vi "Parameters.vi"() -> ()   [LabVIEW 2020, in "Parameters Lib.lvlib"]
uses:
  Parameters Lib.lvlib
  Database Lib.lvlib
panel:
  in  "Reject Based on":string(combo)
  in  "Maximum Area (mm)":i32
  in  "Maximum Length (mm)":i32
  in  "Maximum Width (mm)":i32
  in  "Close":bool
  # "Parameters"
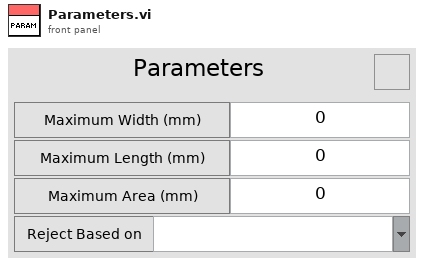
[diagram p1: front panel]
types:
  T1 = cluster{"Maximum Width (mm)":i32, "Maximum Length (mm)":i32, "Maximum Area (mm)":i32, "Reject Based on":string}
  T2 = cluster{"Maximum Width (mm)":i32, "Maximum Length (mm)":i32, "Maximum Area (mm)":i32, "Reject Based on":string}[]
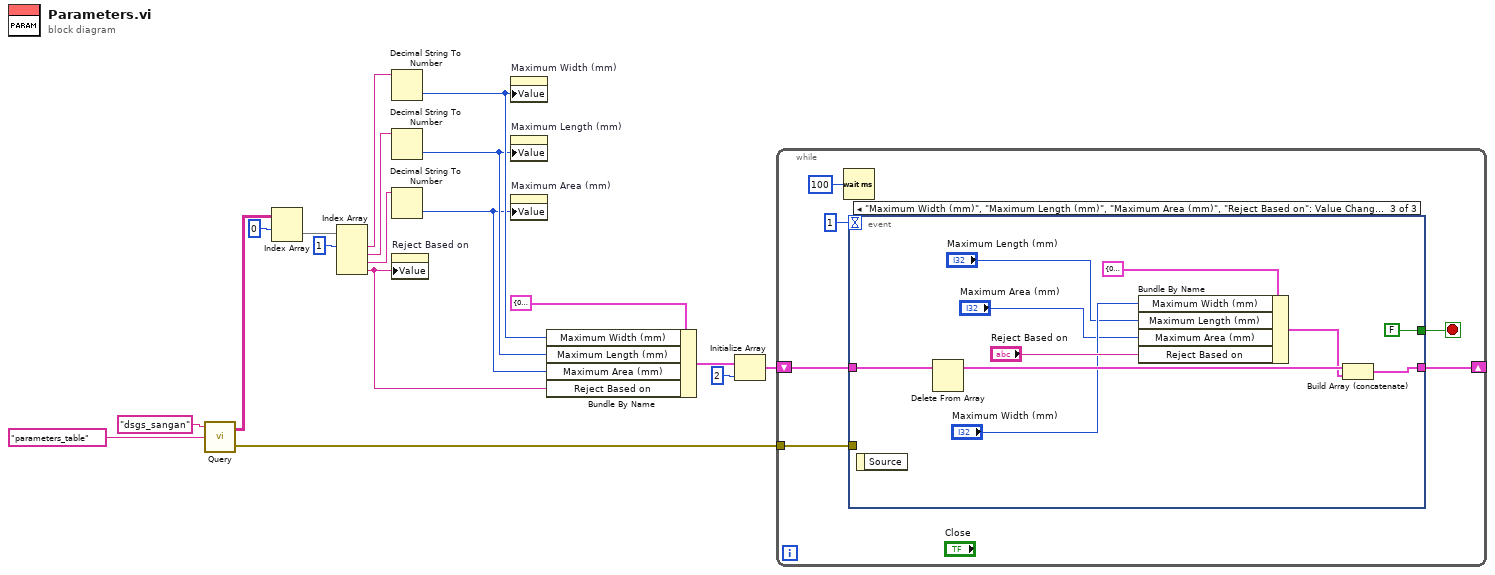
[diagram p0: block diagram]
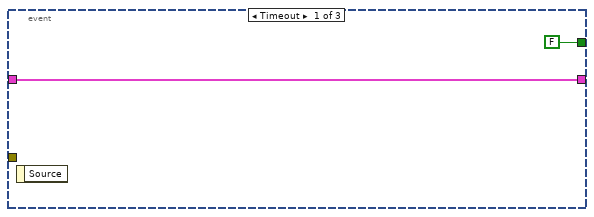
[diagram p2: hidden frame]
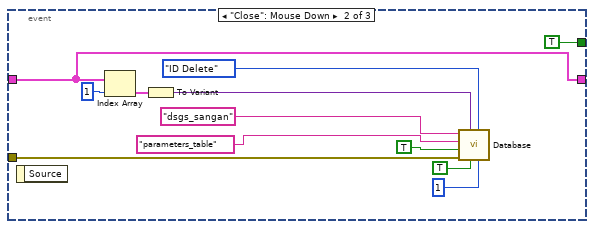
[diagram p3: hidden frame]
diagram:
  n1 = call "Query.vi"("Table Name"="parameters_table" ("Table"), "Connection Name"="dsgs_sangan") -> ("Error out"=w14:errorcluster, "data"=w13:string[][])  [unwired: 2 in]
  n2 = Index Array(array=w13, index (row)=0) -> (element=w11:string[])  [unwired: 1 in]
  n3 = Index Array(array=w11, index #1=1 ("index")) -> (element #1=w8:string, element #2=w6:string, element #3=w7:string, element #4=w1:string)  [unwired: 3 in]
  n4 = Decimal String To Number(string=w8) -> (number=w4:i32)  [unwired: 2 in, 1 out]
  n5 = Decimal String To Number(string=w6) -> (number=w3:i32)  [unwired: 2 in, 1 out]
  n6 = Decimal String To Number(string=w7) -> (number=w2:i32)  [unwired: 2 in, 1 out]
  n7 = property on="Reject Based on" class="CmbBox"("Value"=w1) -> ()  [unwired: 2 in, 2 out]
  n8 = property on="Maximum Width (mm)" class="DigNum (strict)"("Value"=w4) -> ()  [unwired: 2 in, 2 out]
  n9 = property on="Maximum Length (mm)" class="DigNum (strict)"("Value"=w3) -> ()  [unwired: 2 in, 2 out]
  n10 = property on="Maximum Area (mm)" class="DigNum (strict)"("Value"=w2) -> ()  [unwired: 2 in, 2 out]
  n11 = Bundle By Name(cluster=T1 {"Maximum Width (mm)"=0, "Maximum Length (mm)"=0, "Maximum Area (mm)"=0, "Reject Based on"=""}, "Maximum Width (mm)"=w4, "Maximum Length (mm)"=w3, "Maximum Area (mm)"=w2, "Reject Based on"=w1) -> (w9:T1)
  n12 = Initialize Array(w9, 2 ("dimension size")) -> (w18:T2)
  n13 = while {
    shift-right: [w20] -> _
    shift-left: w18 -> [w21]
    tunnel: w14 -> [w19]
    stop <- w23 stop-if-true
    n14 = Wait (ms)(milliseconds to wait=u32 100) -> ()  [unwired: 1 out]
    n15 = event shown="[2] \"Maximum Width (mm)\", \"Maximum Length (mm)\", \"Maximum Area (mm)\", \"Reject Based on\": Value Change" {
      selector: _ -> [_ _ _]
      dyn-events: _ -> [_ _ _]
      timeout: 1 -> [_ _ _]
      tunnel: [FALSE TRUE FALSE] -> w23
      tunnel: w21 -> [w25 w30 w47]
      tunnel: [w25 w30 w41] -> w20
      tunnel: w19 -> [_ w27 _]
      event Timeout {
        n16 = event-data() -> ()  [unwired: 1 in, 1 out]
      }
      event "Close": Mouse Down {
        n17 = event-data() -> ()  [unwired: 1 in, 1 out]
        n18 = Index Array(array=w30, index=1) -> (element=w28:T1)
        n19 = To Variant(anything=w28) -> (Variant=w31:variant)
        n20 = call "Database.vi"("Maximum Row"=1, "Enum"=enum16{"ID Delete", "Time Delete"}."ID Delete", "Delete row?"=TRUE, "Data"=w31, "Error in"=w27, "Auto Increment ID?"=TRUE, "Table"="parameters_table", "Connection"="dsgs_sangan") -> ()  [unwired: 3 in, 1 out]
      }
      event "Maximum Width (mm)", "Maximum Length (mm)", "Maximum Area (mm)", "Reject Based on": Value Change {
        n21 = event-data() -> ()  [unwired: 1 in, 1 out]
        n22 = Delete From Array(array=w47) -> (array with subset deleted=w46:T2)  [unwired: 2 in, 1 out]
        n23 = Bundle By Name(cluster=T1 {"Maximum Width (mm)"=0, "Maximum Length (mm)"=0, "Maximum Area (mm)"=0, "Reject Based on"=""}, "Maximum Width (mm)"="Maximum Width (mm)", "Maximum Length (mm)"="Maximum Length (mm)", "Maximum Area (mm)"="Maximum Area (mm)", "Reject Based on"="Reject Based on") -> (w40:T1)
        n24 = Build Array (concatenate)(w46, w40) -> (w41:T2)
      }
    }
  }
